vi "Savitzky-Golay Filtering.vi"() -> ()   [LabVIEW 2023]
doc: "This example demonstrates how to use the Savitzky-Golay Filter VI to design a Savitzky-Golay filter and use it to smooth a noisy signal."
uses:
  <vilib>/Analysis/3filter.llb/Savitzky-Golay Filter (DBL).vi
  <vilib>/Analysis/NI_AALBase.lvlib
panel:
  in  "seed":i32=-1
  in  "Stop":bool
  out "Waveform Graph":dbl[][](graph)
  in  "samples":i32=300
  in  "polynomial order":i32(slide)=3 scale=0.0..20.0
  in  "side points":i32(slide)=24 scale=0.0..40.0
  # "Overview: Demonstrates how to use the Savitzky-Golay Filter VI to smooth a noisy signal.\nRequirements: LabVIEW Full Development System\nInstructions:\n1. Run the VI to see the noisy and smoothed signals.\n2. Modify the side points and polynomial order.\n3. Change the seed value to generate different noise values.\n4. Click Stop to stop the VI."
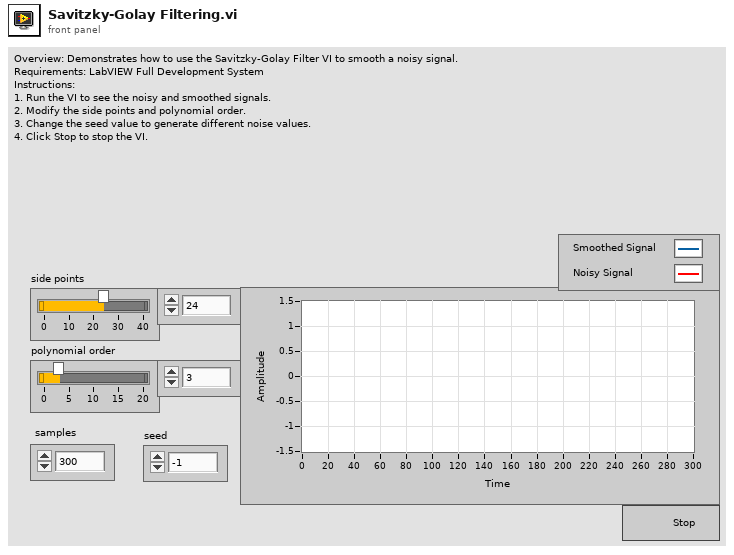
[diagram p1: front panel]
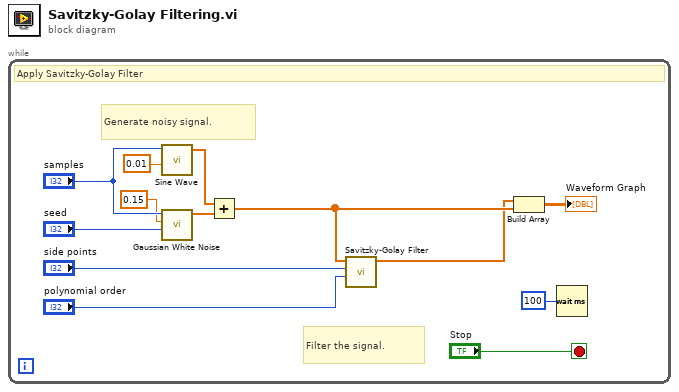
[diagram p0: block diagram]
diagram:
  n1 = while {
    stop <- "Stop" stop-if-true
    # "Filter the signal."
    # "Generate noisy signal."
    # "Apply Savitzky-Golay Filter"
    n2 = call <vilib>:"Sine Wave.vi"("samples"="samples", "frequency"=0.01 ("f")) -> ("sine wave"=w10:dbl[])  [unwired: 3 in, 2 out]
    n3 = call <vilib>:"Gaussian White Noise.vi"("seed"="seed", "standard deviation"=0.15, "samples"="samples") -> ("Gaussian noise pattern"=w9:dbl[])  [unwired: 7 in, 1 out]
    n4 = Add(x=w10, y=w9) -> (x+y=w6:dbl[])
    n5 = call-poly <vilib>:"Savitzky-Golay Filter.vi"("polynomial order"="polynomial order", "side points"="side points", "X"=w6) -> ("Filtered X"=w5:dbl[])  [unwired: 7 in, 1 out]
    n6 = Build Array(w5, w6) -> (→"Waveform Graph":dbl[][])
    n7 = Wait (ms)(milliseconds to wait=u32 100) -> ()  [unwired: 1 out]
  }
